vi "MENU_Filters.vi"(3 "Mediated v.":bool, 4 "Offset":dbl=30.0 format="%.1f", 5 "Inversion sign 2":bool=TRUE) -> (0 "Mediated v. 2":bool=TRUE, 1 "Offset 2":dbl, 2 "Inversion sign 3":bool=TRUE caption="Inversion sign 2")   [LabVIEW 2010]
panel:
  in  "Close":bool
  # "FILTERS"
  # "Inv"
  # "Norm"
  # "No"
  # "Yes"
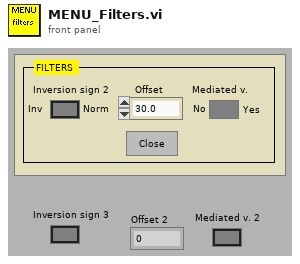
[diagram p1: front panel]
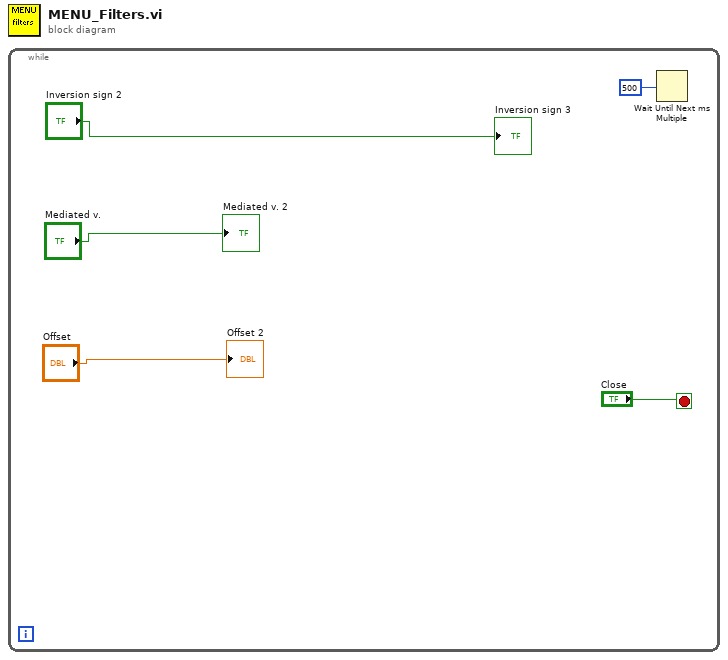
[diagram p0: block diagram]
diagram:
  n1 = while {
    stop <- "Close" stop-if-true
    n2 = Wait Until Next ms Multiple(millisecond multiple=500) -> ()  [unwired: 1 out]
    "Inversion sign 3" <- "Inversion sign 2"
    "Mediated v. 2" <- "Mediated v."
    "Offset 2" <- "Offset"
  }
